vi "PathPlanner_DriveFeedFwds_Flip.vi"(11 "in DriveFeedFwds":T1) -> (3 "flipped DriveFeedFwds":T1)   [LabVIEW 2019, in "PathPlanner24.lvlib"]
doc: "Interpolate between this state and the given state\n \nInputs: \n - trajectoryState - cluster - this trajectory state\n - endVal - cluster - State to interpolate with\n - t - double - Interpolation factor (0.0-1.0)\n\nOutputs:\n - Interpolated state - trajectory state - interpolated state"
uses:
  PathPlanner24.lvlib
  TypeDef/PathPlannerDriveFeedFwds.ctl
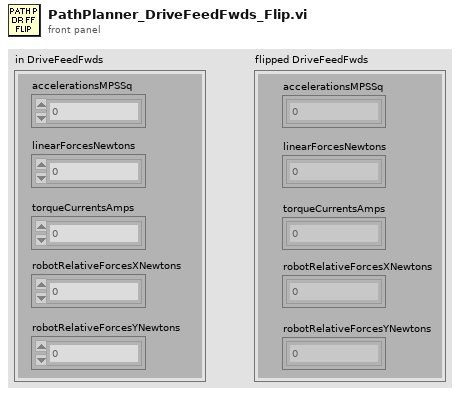
[diagram p1: front panel]
types:
  T1 = typedef "PathPlanner24.lvlib/PathPlannerDriveFeedFwds.ctl" = cluster{"accelerationsMPSSq":dbl[], "linearForcesNewtons":dbl[], "torqueCurrentsAmps":dbl[], "robotRelativeForcesXNewtons":dbl[], "robotRelativeForcesYNewtons":dbl[]}
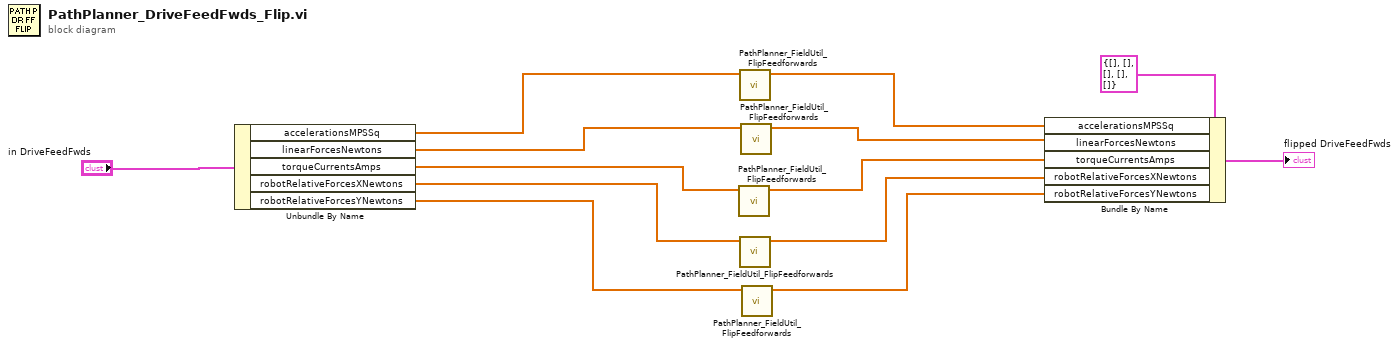
[diagram p0: block diagram]
diagram:
  n1 = Unbundle By Name("in DriveFeedFwds") -> ("accelerationsMPSSq"=w10:dbl[], "linearForcesNewtons"=w9:dbl[], "torqueCurrentsAmps"=w8:dbl[], "robotRelativeForcesXNewtons"=w7:dbl[], "robotRelativeForcesYNewtons"=w6:dbl[])
  n2 = call "PathPlanner_FieldUtil_FlipFeedforwards.vi"("Feedforward"=w8) -> ("FlippedFeedforward"=w3:dbl[])  [unwired: 10 in]
  n3 = call "PathPlanner_FieldUtil_FlipFeedforwards.vi"("Feedforward"=w10) -> ("FlippedFeedforward"=w5:dbl[])  [unwired: 10 in]
  n4 = call "PathPlanner_FieldUtil_FlipFeedforwards.vi"("Feedforward"=w7) -> ("FlippedFeedforward"=w2:dbl[])  [unwired: 10 in]
  n5 = call "PathPlanner_FieldUtil_FlipFeedforwards.vi"("Feedforward"=w9) -> ("FlippedFeedforward"=w4:dbl[])  [unwired: 10 in]
  n6 = call "PathPlanner_FieldUtil_FlipFeedforwards.vi"("Feedforward"=w6) -> ("FlippedFeedforward"=w1:dbl[])  [unwired: 10 in]
  n7 = Bundle By Name(cluster=T1 {"accelerationsMPSSq"=[], "linearForcesNewtons"=[], "torqueCurrentsAmps"=[], "robotRelativeForcesXNewtons"=[], "robotRelativeForcesYNewtons"=[]} ("PathPlannerState"), "accelerationsMPSSq"=w5, "linearForcesNewtons"=w4, "torqueCurrentsAmps"=w3, "robotRelativeForcesXNewtons"=w2, "robotRelativeForcesYNewtons"=w1) -> (→"flipped DriveFeedFwds":T1)
